vi "ReadTemperature.vi"(0 "reference in":refnum<class "BME280.lvclass">, 5 "error in (no error)":errorcluster, 6 "LINX Resource":T1={"IO"=enum."Remote", "Interface"=enum."Serial", "LINX Device Config"={"Interface"=enum."Serial", "COM Port"="COM13", "TCP Configuration"={"IP Address"="", "Port"=0}, "Device Family"=1, "Device ID"=1, "Device Name"="myRIO-1900", "TCP Ref"=refnum, "Channels"={"DI"=[0, 1, 2, 3, 4, 5, 6, 7, 8, 9, 10, 11, 12, 13, 14, 15, 16, 17, 18, 19, 20, 21, 22, 23, 24, 25, 26, 27, 28, 29, 30, 31, 32, 33, 34, 35, 36, 37, 38, 39, 40, 41, 42, 43, 44, 45, 46], "DO"=[0, 1, 2, 3, 4, 5, 6, 7, 8, 9, 10, 11, 12, 13, 14, 15, 16, 17, 18, 19, 20, 21, 22, 23, 24, 25, 26, 27, 28, 29, 30, 31, 32, 33, 34, 35, 36, 37, 38, 39, 40, 41, 42, 43, 44, 45, 46], "AI"=[0, 1, 2, 3, 4, 5, 6, 7, 8, 9, 10, 11], "AO"=[], "PWM"=[3, 5, 6, 9, 10], "QE"=[], "UART"=[0, 1], "I2C 2"=[0], "SPI"=[0], "CAN"=[], "Servo"=[], "AI Ref (V)"=0.0, "AI Resolution (Bits)"=0, "AO Ref (V)"=0.0, "AO Resolution (Bits)"=0}}}, 8 "I2C Channel (0)":u8=1) -> (12 "LINX Resource":T1={"IO"=enum."Remote", "Interface"=enum."Serial", "LINX Device Config"={"Interface"=enum."Serial", "COM Port"="COM13", "TCP Configuration"={"IP Address"="", "Port"=0}, "Device Family"=1, "Device ID"=1, "Device Name"="myRIO-1900", "TCP Ref"=refnum, "Channels"={"DI"=[0, 1, 2, 3, 4, 5, 6, 7, 8, 9, 10, 11, 12, 13, 14, 15, 16, 17, 18, 19, 20, 21, 22, 23, 24, 25, 26, 27, 28, 29, 30, 31, 32, 33, 34, 35, 36, 37, 38, 39, 40, 41, 42, 43, 44, 45, 46], "DO"=[0, 1, 2, 3, 4, 5, 6, 7, 8, 9, 10, 11, 12, 13, 14, 15, 16, 17, 18, 19, 20, 21, 22, 23, 24, 25, 26, 27, 28, 29, 30, 31, 32, 33, 34, 35, 36, 37, 38, 39, 40, 41, 42, 43, 44, 45, 46], "AI"=[0, 1, 2, 3, 4, 5, 6, 7, 8, 9, 10, 11], "AO"=[], "PWM"=[3, 5, 6, 9, 10], "QE"=[], "UART"=[0, 1], "I2C 2"=[0], "SPI"=[0], "CAN"=[], "Servo"=[], "AI Ref (V)"=0.0, "AI Resolution (Bits)"=0, "AO Ref (V)"=0.0, "AO Resolution (Bits)"=0}}}, 14 "reference out":refnum<class "BME280.lvclass">, 15 "Temperature":dbl, 17 "Data Temp":u8[](array[numeric]), 19 "error out":errorcluster)   [LabVIEW 2014, in "BME280.lvclass"]
uses:
  BME280.lvclass
  <vilib>/MakerHub/LINX/Private/Type Defs/LINX Ref.ctl
  <vilib>/MakerHub/LINX/Private/Type Defs/Platform.ctl
  <vilib>/MakerHub/LINX/Private/Type Defs/Interface.ctl
  <vilib>/MakerHub/LINX/Private/Device/Type Defs/LINX Device Config.ctl
  <vilib>/MakerHub/LINX/Private/Device/Type Defs/TCP Config.ctl
  <vilib>/MakerHub/LINX/Private/Device/Type Defs/Channels.ctl
  <vilib>/MakerHub/LINX/Private/Local IO/LinxI2cWrite.vi
  <vilib>/MakerHub/LINX/Public/Utilities/Check Channel.vi
  <vilib>/MakerHub/LINX/Private/Local IO/Handle Errors.vi
  <vilib>/MakerHub/LINX/Private/Utilties/Generate Error.vi
  <vilib>/MakerHub/LINX/LMH-LINX.lvlib
  <vilib>/MakerHub/LINX/Private/Device/Device.lvlib
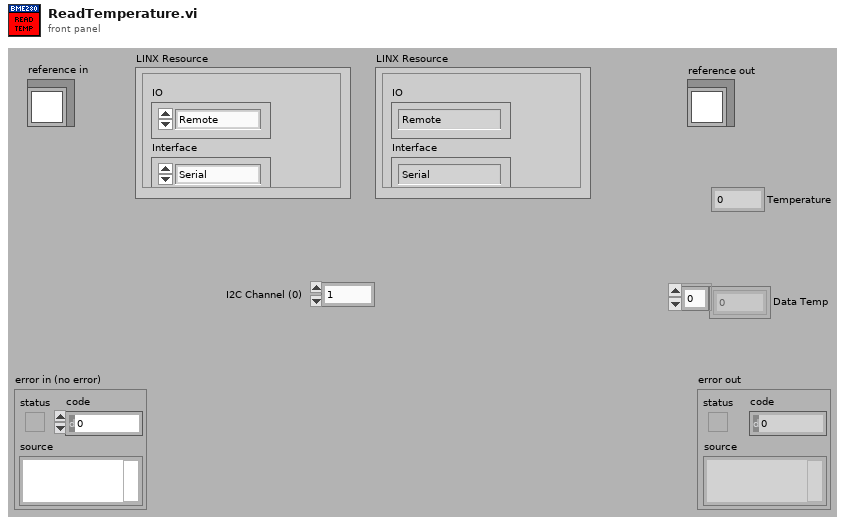
[diagram p1: front panel]
types:
  T1 = typedef "LMH-LINX.lvlib/LINX Ref.ctl" = cluster{"IO":T2, "Interface":T3, "LINX Device Config":T4}
  T2 = typedef "LMH-LINX.lvlib/Platform.ctl" = enum16{"Remote", "Local"}
  T3 = typedef "LMH-LINX.lvlib/Interface.ctl" = enum16{"Serial", "TCP"}
  T4 = typedef "LMH-LINX.lvlib/Device.lvlib/LINX Device Config.ctl" = cluster{"Interface":T3, "COM Port":refnum<visa-resource-name>, "TCP Configuration":T5, "Device Family":u8, "Device ID":u8, "Device Name":string, "TCP Ref":refnum<k5>, "Channels":T6}
  T5 = typedef "LMH-LINX.lvlib/Device.lvlib/TCP Config.ctl" = cluster{"IP Address":string, "Port":u16}
  T6 = typedef "LMH-LINX.lvlib/Channels.ctl" = cluster{"DI":u8[], "DO":u8[], "AI":u8[], "AO":u8[], "PWM":u8[], "QE":u8[], "UART":u8[], "I2C 2":u8[], "SPI":u8[], "CAN":u8[], "Servo":u8[], "AI Ref (V)":dbl, "AI Resolution (Bits)":u8, "AO Ref (V)":dbl, "AO Resolution (Bits)":u8}
  T7 = typedef "BME280.lvclass/ObjectAttributes.ctl" = cluster{"I2C Slave Address":u8, "TrimmingParameters":T8, "t_fine":i32}
  T8 = typedef "BME280.lvclass/TrimmingParameters.ctl" = cluster{"dig_T1":u16, "dig_T2":i16, "dig_T3":i16, "dig_P1":u16, "dig_P2":i16, "dig_P3":i16, "dig_P4":i16, "dig_P5":i16, "dig_P6":i16, "dig_P7":i16, "dig_P8":i16, "dig_P9":i16, "dig_H1":u8, "dig_H2":i16, "dig_H3":u8, "dig_H4":i16, "dig_H5":i16, "dig_H6":i8}
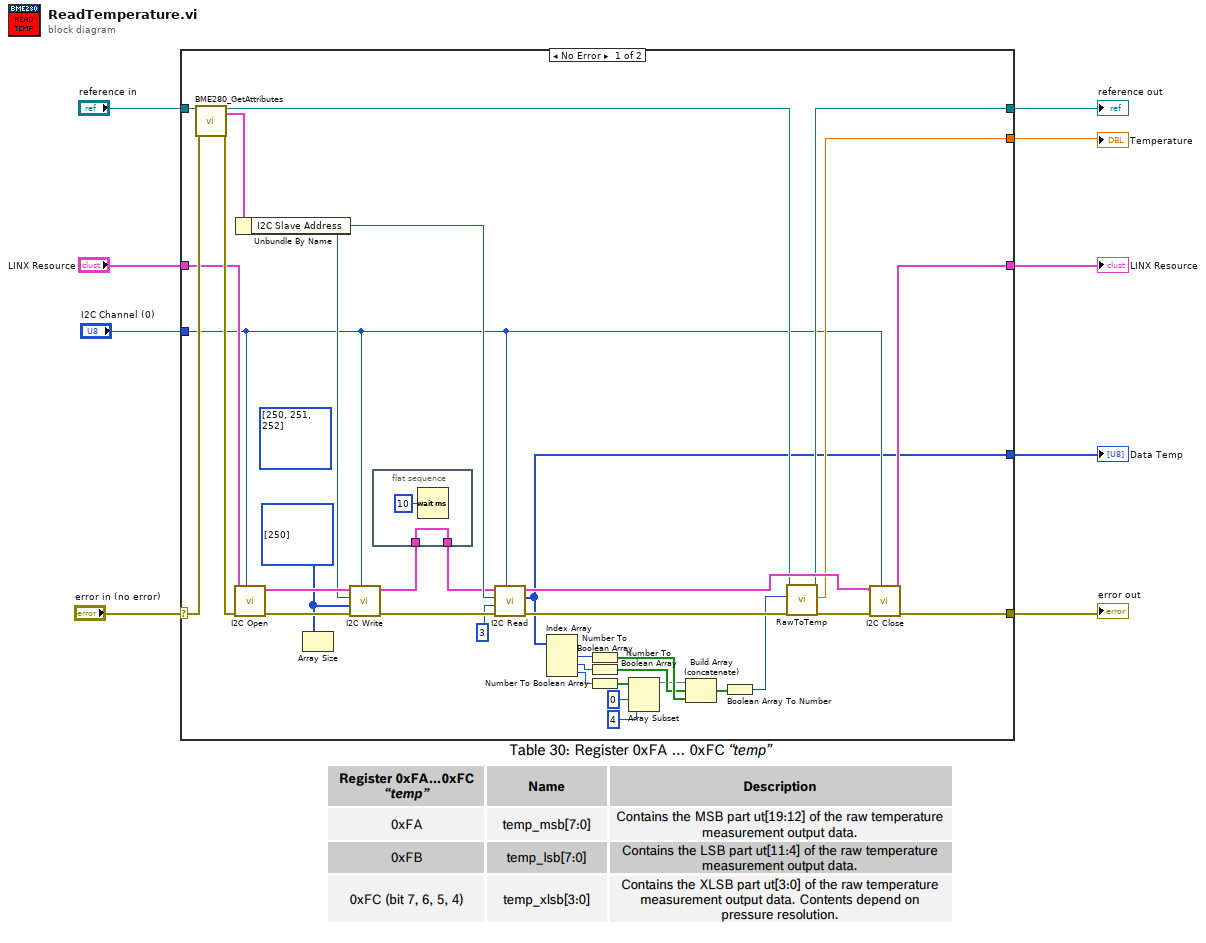
[diagram p0: block diagram]
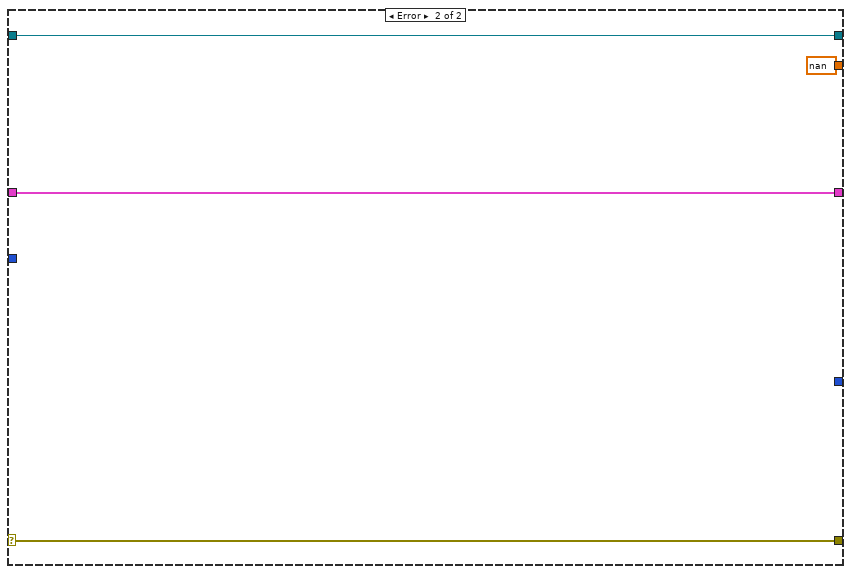
[diagram p2: hidden frame]
diagram:
  n1 = case shown="No Error" "error in (no error)" {
    selector: "error in (no error)" -> [w43 w49]
    tunnel: [w39 w49] -> w8
    tunnel: [w26 w48] -> w6
    tunnel: "reference in" -> [w42 w48]
    tunnel: "LINX Resource" -> [w40 w47]
    tunnel: [w38 w47] -> w4
    tunnel: [w25 nan] -> w3
    tunnel: [w23 _] -> w2
    tunnel: "I2C Channel (0)" -> [w24 _]
    frame No Error {
      w10 = u8[] [250] ("Data")
      (unwired) u8[] [250, 251, 252] ("Data")
      n2 = call "BME280_GetAttributes.vi"("reference in"=w42, "error in (no error)"=w43) -> ("reference out"=w27:refnum<class "BME280.lvclass">, "Data"=w37:T7, "error out"=w41:errorcluster)  [unwired: 14 in, 1 out]
      n3 = call <vilib>:"I2C Open.vi"("I2C Channel (0)"=w24, "Error In"=w41, "LINX Resource"=w40) -> ("Error Out"=w30:errorcluster, "LINX Resource"=w36:T1)  [unwired: 7 in]
      n4 = Unbundle By Name(w37) -> ("I2C Slave Address"=w34:u8)
      n5 = Array Size(array=w10) -> ()  [unwired: 1 out]
      n6 = call <vilib>:"I2C Write.vi"("I2C Channel"=w24, "Error In"=w30, "Data"=w10, "I2C Slave Address (0)"=w34, "LINX Resource"=w36) -> ("Error Out"=w35:errorcluster, "LINX Resource"=w32:T1)  [unwired: 5 in]
      n7 = flat-sequence {
        tunnel: [w45] -> w31
        tunnel: w32 -> [w45]
        frame #0 {
          n8 = Wait (ms)(milliseconds to wait=u32 10) -> ()  [unwired: 1 out]
        }
      }
      n9 = call <vilib>:"I2C Read.vi"("I2C Channel"=w24, "Error In"=w35, "Bytes To Read"=u8 3, "I2C Slave Address (0)"=w34, "LINX Resource"=w31) -> ("Error Out"=w29:errorcluster, "Data"=w23:u8[], "LINX Resource"=w33:T1)  [unwired: 4 in]
      n10 = Index Array(array=w23) -> (element #1=w22:u8, element #2=w21:u8, element #3=w20:u8)  [unwired: 3 in]
      n11 = Number To Boolean Array(number=w22) -> (Boolean array=w19:bool[])
      n12 = Number To Boolean Array(number=w21) -> (Boolean array=w18:bool[])
      n13 = Number To Boolean Array(number=w20) -> (Boolean array=w17:bool[])
      n14 = Array Subset(array=w17, index=0, length=4) -> (w16:bool[])
      n15 = Build Array (concatenate)(w16, w18, w19) -> (w13:bool[])
      n16 = Boolean Array To Number(Boolean array=w13) -> (number=w12:u32)
      n17 = call "RawToTemp.vi"("reference in"=w27, "T_ADC"=w12, "error in (no error)"=w29) -> ("reference out"=w26:refnum<class "BME280.lvclass">, "T"=w25:dbl, "error out"=w28:errorcluster)  [unwired: 14 in]
      n18 = call <vilib>:"I2C Close.vi"("I2C Channel (0)"=w24, "Error In"=w28, "LINX Resource"=w33) -> ("Error Out"=w39:errorcluster, "LINX Resource"=w38:T1)  [unwired: 7 in]
    }
    frame Error {
    }
  }
  "error out" <- w8
  "reference out" <- w6
  "LINX Resource" <- w4
  "Temperature" <- w3
  "Data Temp" <- w2
